vi "Tank_4_Motor.vi"(8 "Front Right Motor":T3={"DeviceStatus"={"status"=FALSE, "code"=0, "source"=""}, "Type"=enum."PWM", "PWM"={"PWM Channel"=enum."Invalid", "DeadBand"={"Name"="", "maxPositivePwm"=0, "minPositivePwm"=0, "centerPwm"=0, "maxNegativePwm"=0, "minNegativePwm"=0, "angularRange"=0}}, "CAN"={"Device Number"=0, "SetOutput VI Ref"=variant(refnum<vi> refnum), "GetOutput VI Ref"=variant(refnum<vi> refnum), "Enable VI Ref"=variant(refnum<vi> refnum), "Disable VI Ref"=variant(refnum<vi> refnum), "Data"=variant}, "Invert"=FALSE}, 9 "Front Left Motor":T3={"DeviceStatus"={"status"=FALSE, "code"=0, "source"=""}, "Type"=enum."PWM", "PWM"={"PWM Channel"=enum."Invalid", "DeadBand"={"Name"="", "maxPositivePwm"=0, "minPositivePwm"=0, "centerPwm"=0, "maxNegativePwm"=0, "minNegativePwm"=0, "angularRange"=0}}, "CAN"={"Device Number"=0, "SetOutput VI Ref"=variant(refnum<vi> refnum), "GetOutput VI Ref"=variant(refnum<vi> refnum), "Enable VI Ref"=variant(refnum<vi> refnum), "Disable VI Ref"=variant(refnum<vi> refnum), "Data"=variant}, "Invert"=FALSE}, 10 "Rear Right Motor":T3={"DeviceStatus"={"status"=FALSE, "code"=0, "source"=""}, "Type"=enum."PWM", "PWM"={"PWM Channel"=enum."Invalid", "DeadBand"={"Name"="", "maxPositivePwm"=0, "minPositivePwm"=0, "centerPwm"=0, "maxNegativePwm"=0, "minNegativePwm"=0, "angularRange"=0}}, "CAN"={"Device Number"=0, "SetOutput VI Ref"=variant(refnum<vi> refnum), "GetOutput VI Ref"=variant(refnum<vi> refnum), "Enable VI Ref"=variant(refnum<vi> refnum), "Disable VI Ref"=variant(refnum<vi> refnum), "Data"=variant}, "Invert"=FALSE}, 11 "Rear Left Motor":T3={"DeviceStatus"={"status"=FALSE, "code"=0, "source"=""}, "Type"=enum."PWM", "PWM"={"PWM Channel"=enum."Invalid", "DeadBand"={"Name"="", "maxPositivePwm"=0, "minPositivePwm"=0, "centerPwm"=0, "maxNegativePwm"=0, "minNegativePwm"=0, "angularRange"=0}}, "CAN"={"Device Number"=0, "SetOutput VI Ref"=variant(refnum<vi> refnum), "GetOutput VI Ref"=variant(refnum<vi> refnum), "Enable VI Ref"=variant(refnum<vi> refnum), "Disable VI Ref"=variant(refnum<vi> refnum), "Data"=variant}, "Invert"=FALSE}) -> (3 "DriveCluster_Out":T1={"Valid Commands"=[], "RobotDriveDevRef"={"DevStatus"={"status"=FALSE, "code"=0, "source"=""}, "Motors[]"=[], "Square Inputs"=FALSE, "Max Output"=1.0}, "Drive Train"=enum."Tank Drive 2 Motor"})   [LabVIEW 2016]
uses:
  <vilib>/Rock Robotics/WPI/MotorControl/WPI_MotorControlDeviceRef.ctl
  <vilib>/Rock Robotics/WPI/MotorControl/WPI_MotorControlType.ctl
  <vilib>/Rock Robotics/SystemInterfaces/DIO/FPGA_DIOPWMChannel.ctl
  <vilib>/Rock Robotics/WPI/PWM/WPI_PWMDeadband.ctl
  <userlib>/836-libraries/Drive/Drive_Code_V2/Drive_Code_Support/Drive_Reference.ctl
  <vilib>/Rock Robotics/WPI/RobotDrive/WPI_RobotDriveDevRef.ctl
  <userlib>/836-libraries/Drive/Drive_Code_V2/Drive_Code_Support/Drive_Trains.ctl
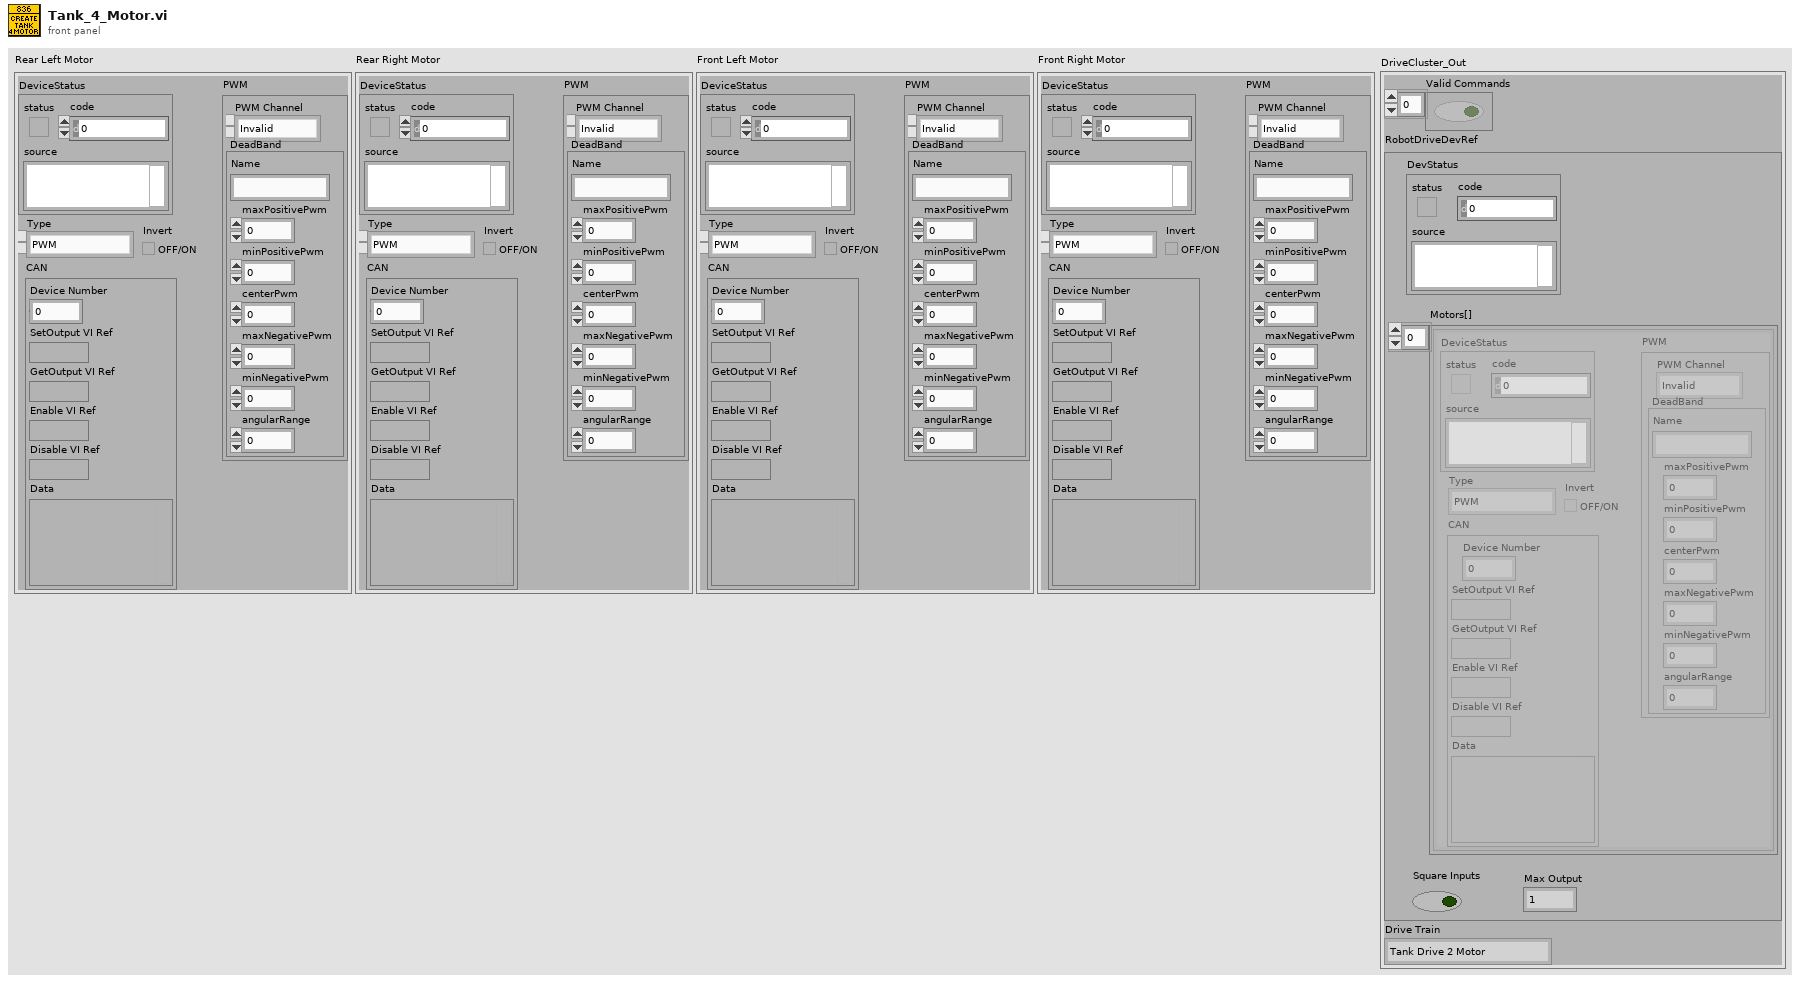
[diagram p1: front panel]
types:
  T1 = typedef "Drive_Reference.ctl" = cluster{"Valid Commands":bool[], "RobotDriveDevRef":T2, "Drive Train":T7}
  T2 = typedef "WPI_RobotDriveDevRef.ctl" = cluster{"DevStatus":errorcluster, "Motors[]":T3[], "Square Inputs":bool, "Max Output":dbl}
  T3 = typedef "WPI_MotorControlDeviceRef.ctl" = cluster{"DeviceStatus":errorcluster, "Type":T4, "PWM":cluster{"PWM Channel":T5, "DeadBand":T6}, "CAN":cluster{"Device Number":u8, "SetOutput VI Ref":variant, "GetOutput VI Ref":variant, "Enable VI Ref":variant, "Disable VI Ref":variant, "Data":variant}, "Invert":bool}
  T4 = typedef "WPI_MotorControlType.ctl" = enum16{"PWM", "CAN"}
  T5 = typedef "FPGA_DIOPWMChannel.ctl" = enum8{"PWM 0", "PWM 1", "PWM 2", "PWM 3", "PWM 4", "PWM 5", "PWM 6", "PWM 7", "PWM 8", "PWM 9", "PWM MXP 0", "PWM MXP 1", "PWM MXP 2", "PWM MXP 3", "PWM MXP 4", "PWM MXP 5", "PWM MXP 6", "PWM MXP 7", "PWM MXP 8", "PWM MXP 9", "Invalid"}
  T6 = typedef "WPI_PWMDeadband.ctl" = cluster{"Name":string, "maxPositivePwm":i32, "minPositivePwm":i32, "centerPwm":i32, "maxNegativePwm":i32, "minNegativePwm":i32, "angularRange":u16}
  T7 = typedef "Drive_Trains.ctl" = enum16{"Tank Drive 2 Motor", "Tank Drive 4 Motor", "Mecanum Drive", "Kiwi Drive"}
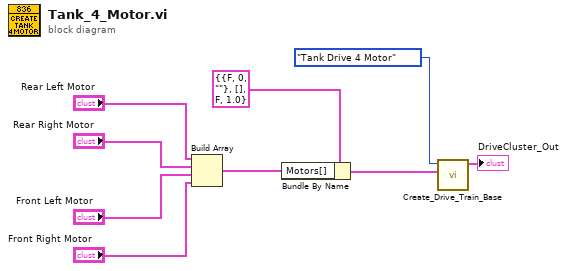
[diagram p0: block diagram]
diagram:
  n1 = Build Array("Rear Left Motor", "Rear Right Motor", "Front Left Motor", "Front Right Motor") -> (w6:T3[])
  n2 = Bundle By Name(cluster=T2 {"DevStatus"={"status"=FALSE, "code"=0, "source"=""}, "Motors[]"=[], "Square Inputs"=FALSE, "Max Output"=1.0} ("RobotDriveDevRef"), "Motors[]"=w6) -> (w5:T2)
  n3 = call <userlib>:"Create_Drive_Train_Base.vi"("RobotDriveDevRef"=w5, "Drive Train"=Drive_Trains."Tank Drive 4 Motor") -> ("DriveCluster_Out"=→"DriveCluster_Out":T1)  [unwired: 9 in]
